vi "project.vi"() -> ()   [LabVIEW 2014]
panel:
  out "Main Valve Position":bool
  out "Motor Running in Delta":bool
  out "Motor Running in Star":bool
  in  "Main Switch Control":bool
  out "Compressor Main Switch":bool
  in  "Boolean":bool
  out "Stage-1 Pressure":u8(slide) scale=0.0..400.0
  out "Inlet Pressure after BDV":u8(slide) scale=0.0..40.0
  out "Inlet\nPressure":u8(slide) scale=0.0..40.0
  out "GD-2 Trend (%LEL)":T1(graph)
  out "GD-1 Trend (%LEL)":T2(graph)
  in  "Low GD-2 %LEL SP":dbl
  in  "High GD-2 %LEL SP":dbl
  in  "Low GD-1 %LEL SP":dbl
  in  "High GD-1 %LEL SP":dbl
  in  "Low Lube Oil Temp SP":dbl
  in  "High Lube Oil Temp SP":dbl
  in  "Low Storage Temp SP":dbl
  in  "High Storage Temp SP":dbl
  in  "Low Stg-3 Temp SP":dbl
  in  "High Stg-3 Temp SP":dbl
  in  "Low Stg-2    Temp SP":dbl
  in  "High Stg-2 Temp SP":dbl
  in  "Low Stg-1 Temp SP":dbl
  in  "High Stg-1 Temp SP":dbl
  in  "Low Inlet Temp SP":dbl
  in  "High Inlet Temp SP":dbl
  in  "Low Lube Oil  Stg-1 Pressure SP":dbl
  in  "High Lube Oil Stg-1 Pressure SP":dbl
  in  "Low Lube Oil Pressure SP":dbl
  in  "High Lube Oil Pressure SP":dbl
  in  "Low Storage Pressure SP":dbl
  in  "High Storage Pressure SP":dbl
  in  "Low Stg-3 Pressure SP 4":dbl
  in  "High Stg-3 Pressure SP":dbl
  in  "Low Stg-2 Pressure SP":dbl
  in  "High Stg-2 Pressure SP":dbl
  in  "Low Stg-1 Pressure SP":dbl
  in  "High Stg-1 Pressure SP":dbl
  in  "Low Inlet Pressure SP":dbl
  in  "High Inlet Pressure SP":dbl
  out "Discharge MFM Flow Rate Trend (Kg/m2)":dbl(graph)
  out "Discharge MFM Total Kg Trend (Kg)":dbl(graph)
  out "Inlet MFM Flow Rate Trend (Kg/m2)":dbl(graph)
  out "Inlet MFM Total Kg Trend (Kg)":dbl(graph)
  out "Lube Oil Temperature Trend (degC)":dbl(graph)
  out "Storage Temperature Trend (degC)":dbl(graph)
  out "Stage-3 Temperature Trend (degC)":dbl(graph)
  out "Stage-2 Temperature Trend (degC)":dbl(graph)
  out "Stage-1 Temperature Trend (degC)":T3(graph)
  out "Inlet Temperature Trend (degC)":T4(graph)
  out "Lube Oil Stage-1 Pressure Trend (Bar) 2":dbl(graph)
  out "Lube Oil Pressure Trend (Bar)":dbl(graph)
  out "Storage Pressure Trend (Bar)":dbl(graph)
  out "Stage-3 Pressure Trend (Bar)":dbl(graph)
  out "Stage-2 Pressure Trend (Bar)":T5(graph)
  out "Stage-1 Pressure Trend (Bar)":T6(graph)
  out "Inlet Pressure after BDV Trend (Bar)":T7(graph)
  out "Inlet Pressure Trend (Bar)":dbl(graph)
  in  "Air Compressor\nstopped/breakdown":bool
  in  "Wire cut":bool
  out "Alarm(s) 4":string
  out "Instrument Air Pressure Gauge (Bar)":dbl(knob) scale=0.0..10.0
  in  "Compressor Start":bool
  out "H":bool
  out "L":bool
  out "H":bool
  out "L":bool
  out "H":bool
  out "L":bool
  out "H":bool
  out "L":bool
  out "H":bool
  out "L":bool
  out "H":bool
  out "L":bool
  out "Alarm(s) 3":string
  out "Alarm(s) 2":string
  out "Lubrication oil Level":dbl(slide) scale=0.0..10.0
  in  "Fill":dbl(slide) scale=0.0..10.0
  out "Alarm(s)":string
  out "CO2 Flooding in Progress":bool
  in  "Fire":bool
  out "Fire Detector-2":bool
  out "Fire Detector-1":bool
  out "Lube Oil Temp":u8(slide) scale=0.0..250.0
  out "Storage Temp":u8(slide) scale=0.0..250.0
  out "Stage-3 \nTemp":u8(slide) scale=0.0..250.0
  out "Stage-2\nTemp":u8(slide) scale=0.0..250.0
  out "Stage-1 \nTemp":u8(slide) scale=0.0..250.0
  out "Inlet\n Temp":u8(slide) scale=0.0..100.0
  out "MFM Flow Rate (Inlet)":dbl
  out "MFM Flow Rate (Discharge)":dbl
  out "MFM Total Kg (Inlet)":dbl format="%#_9g"
  out "MFM Total Kg (Discharge)":dbl format="%#_9g"
  out "Lube oil Stage-1 Pressure":cluster{u8, u8}(slide)={17, 12} scale=0.0..100.0
  out "Lube oil Pressure":cluster{u8, u8}(slide)={17, 12} scale=0.0..10.0
  out "Storage Pressure":cluster{u8, u8}(slide)={17, 12} scale=0.0..400.0
  out "Stage-3 Pressure":cluster{u8, u8}(slide)={17, 12} scale=0.0..400.0
  out "Stage-2 Pressure":cluster{u8, u8}(slide)={17, 12} scale=0.0..400.0
  out "Communication Status":string
  out "Compressor Running Status":string
  # "FIRE SUPPRESSION SAFETY INTERLOCK"
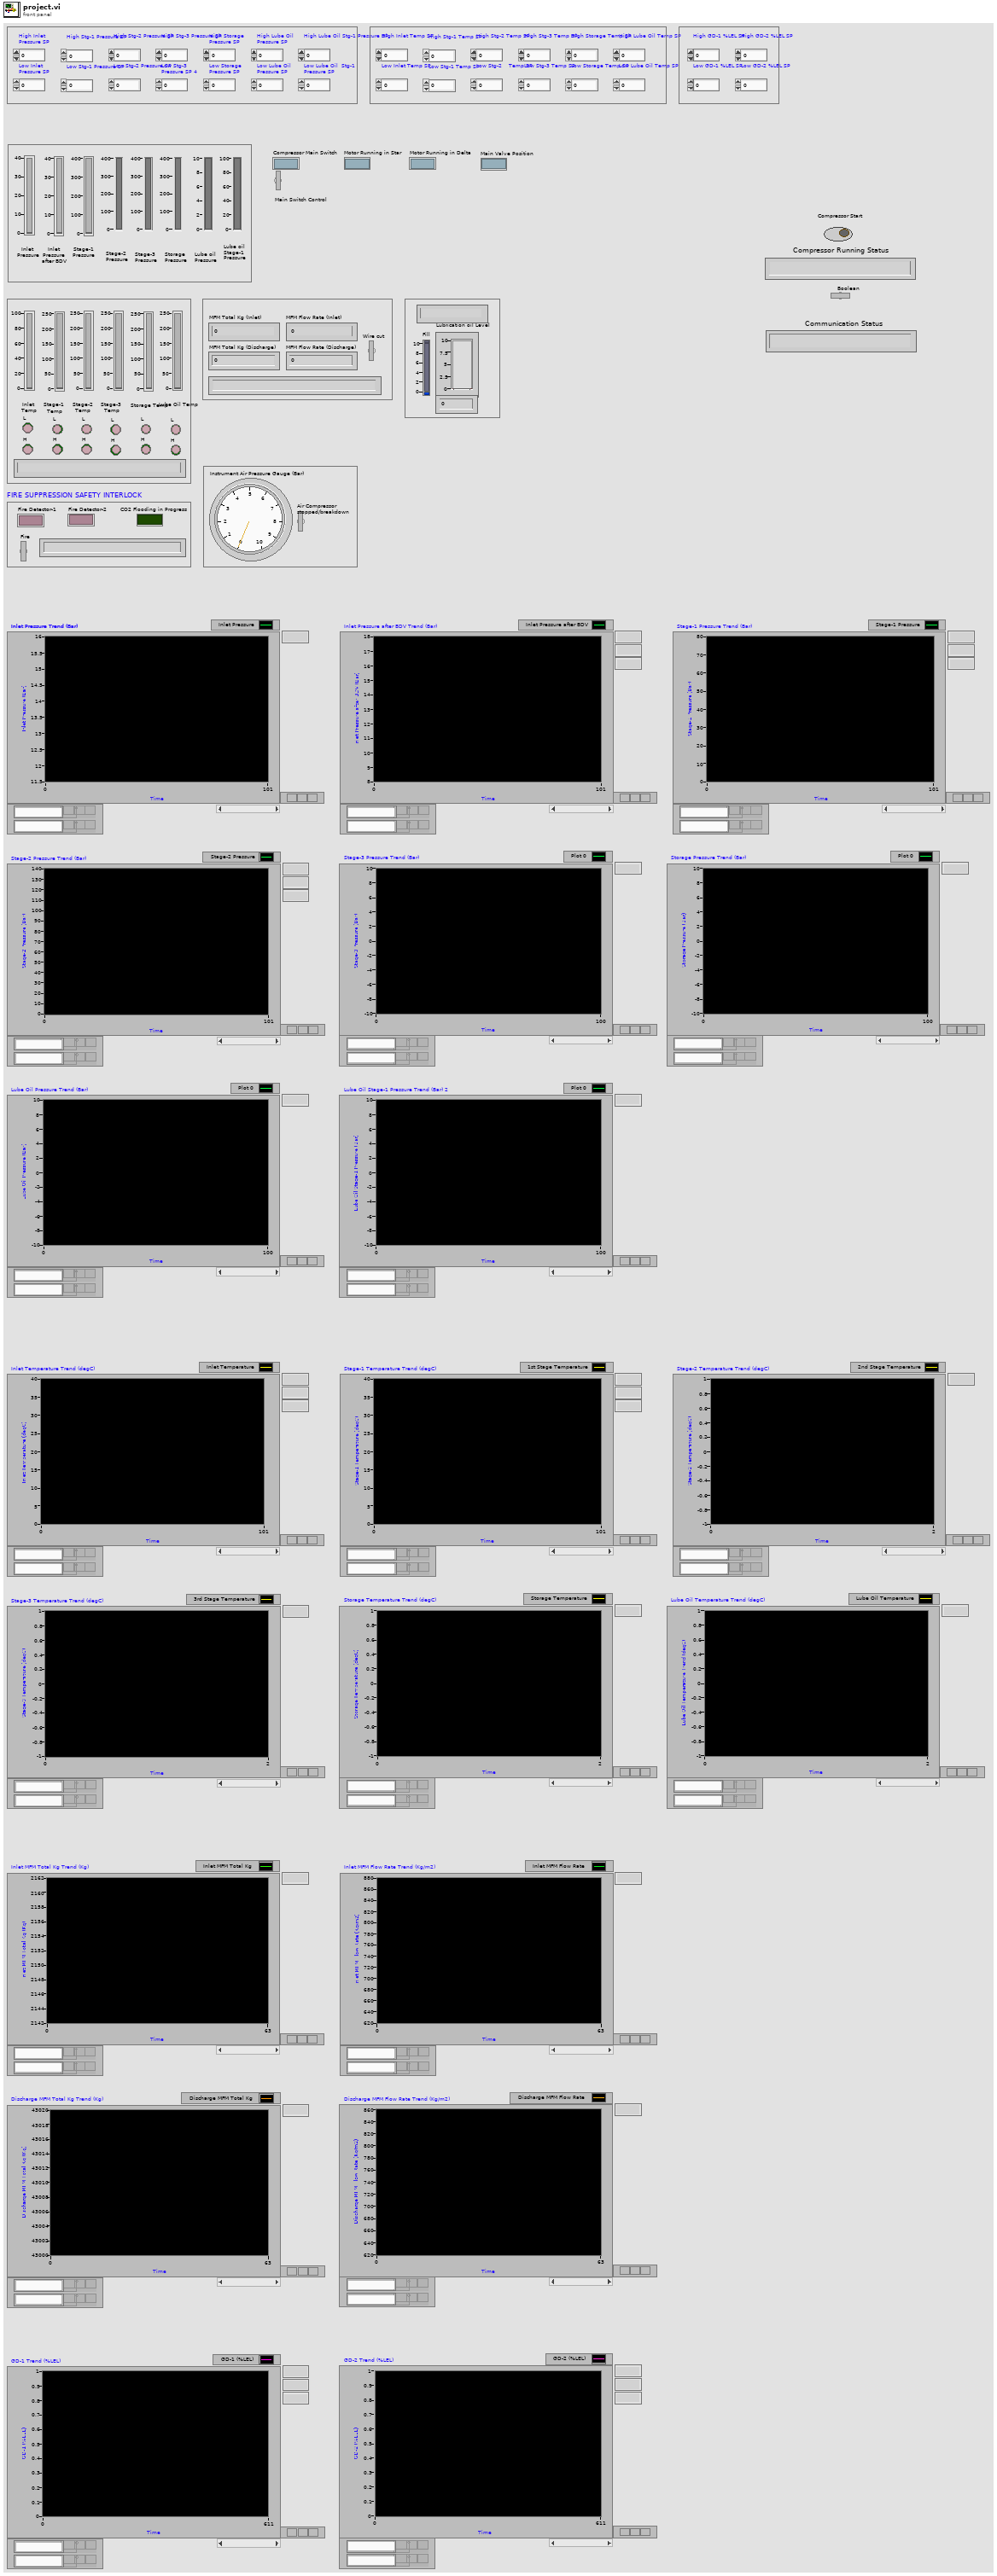
[diagram p1: front panel]
types:
  T1 = cluster{"number: 0 to 1":dbl, "High GD-1 %LEL SP  ":dbl, "Low GD-1 %LEL SP":dbl}
  T2 = cluster{"number: 0 to 1":dbl, "High GD-2 %LEL SP  ":dbl, "Low GD-2 %LEL SP":dbl}
  T3 = cluster{dbl, "High Stg-1 Temp SP":dbl, "Low Stg-1 Temp SP":dbl}
  T4 = cluster{dbl, "High Inlet Temp SP":dbl, "Low Inlet Temp SP":dbl}
  T5 = cluster{dbl, "High Stg-2 Pressure SP":dbl, "Low Stg-2 Pressure SP":dbl}
  T6 = cluster{dbl, "High Stg-1 Pressure SP":dbl, "Low Stg-1 Pressure SP":dbl}
  T7 = cluster{dbl, "High Inlet Pressure SP":dbl, "Low Inlet Pressure SP":dbl}
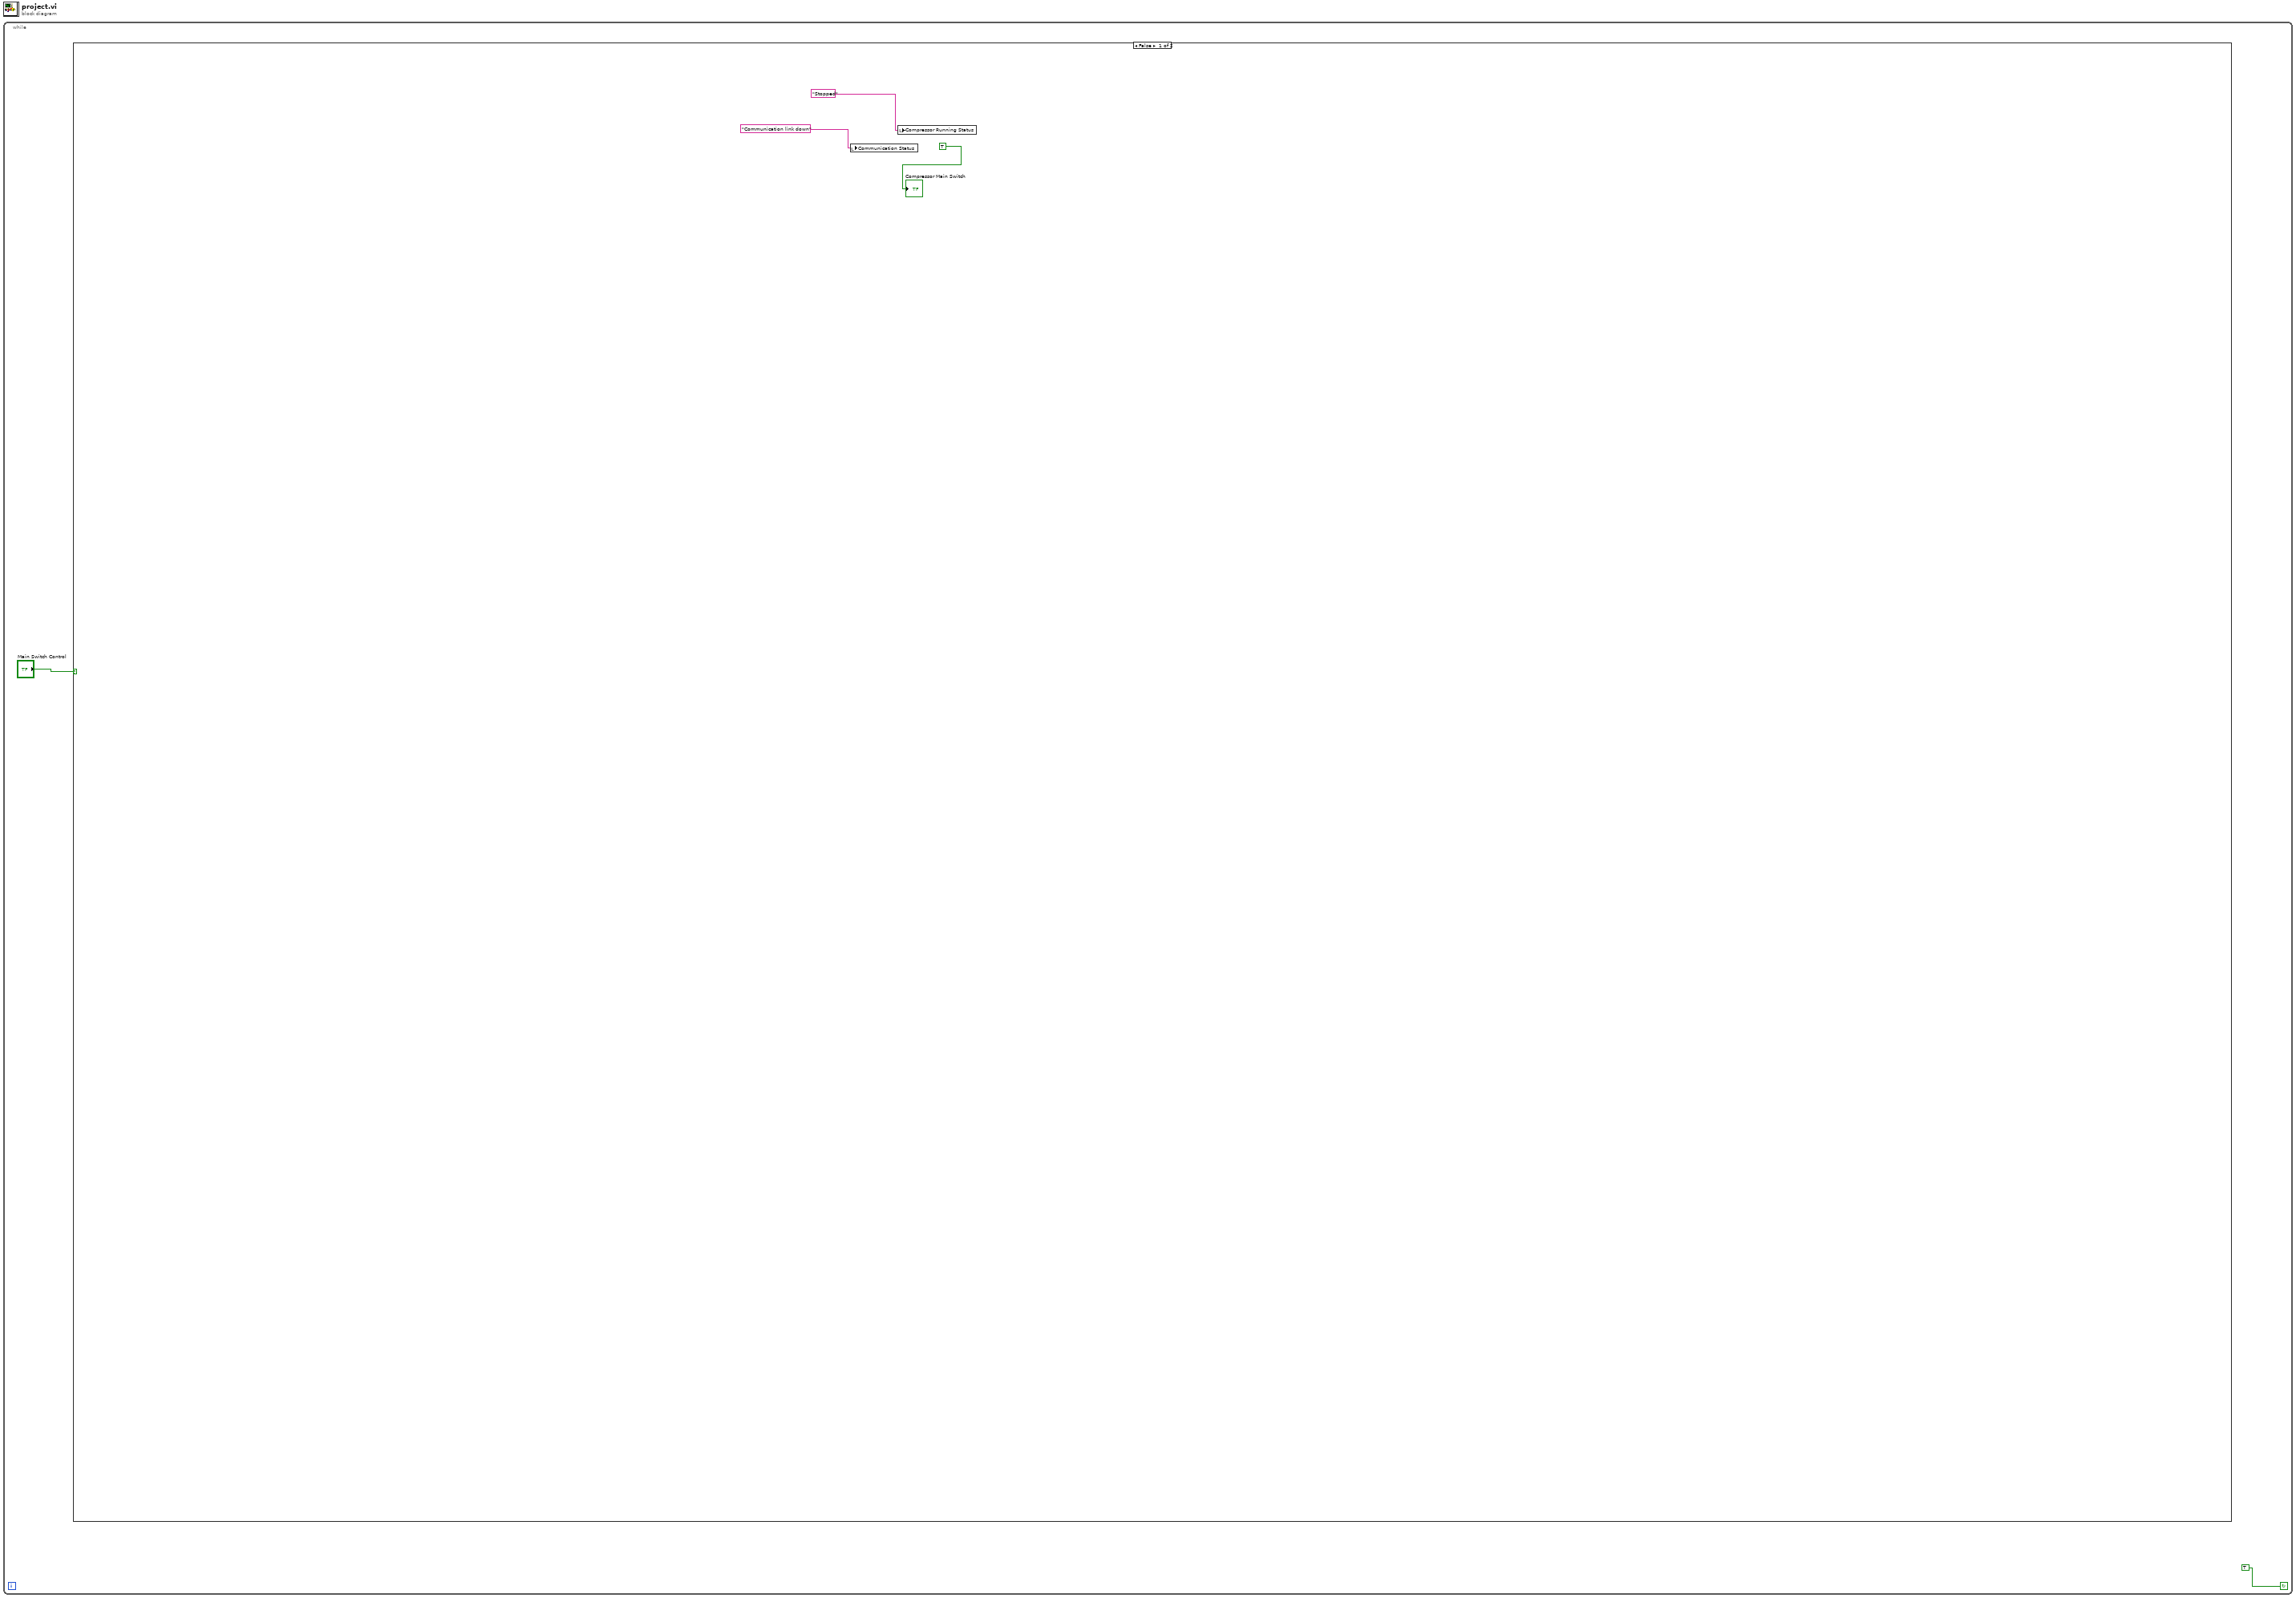
[diagram p0: block diagram]
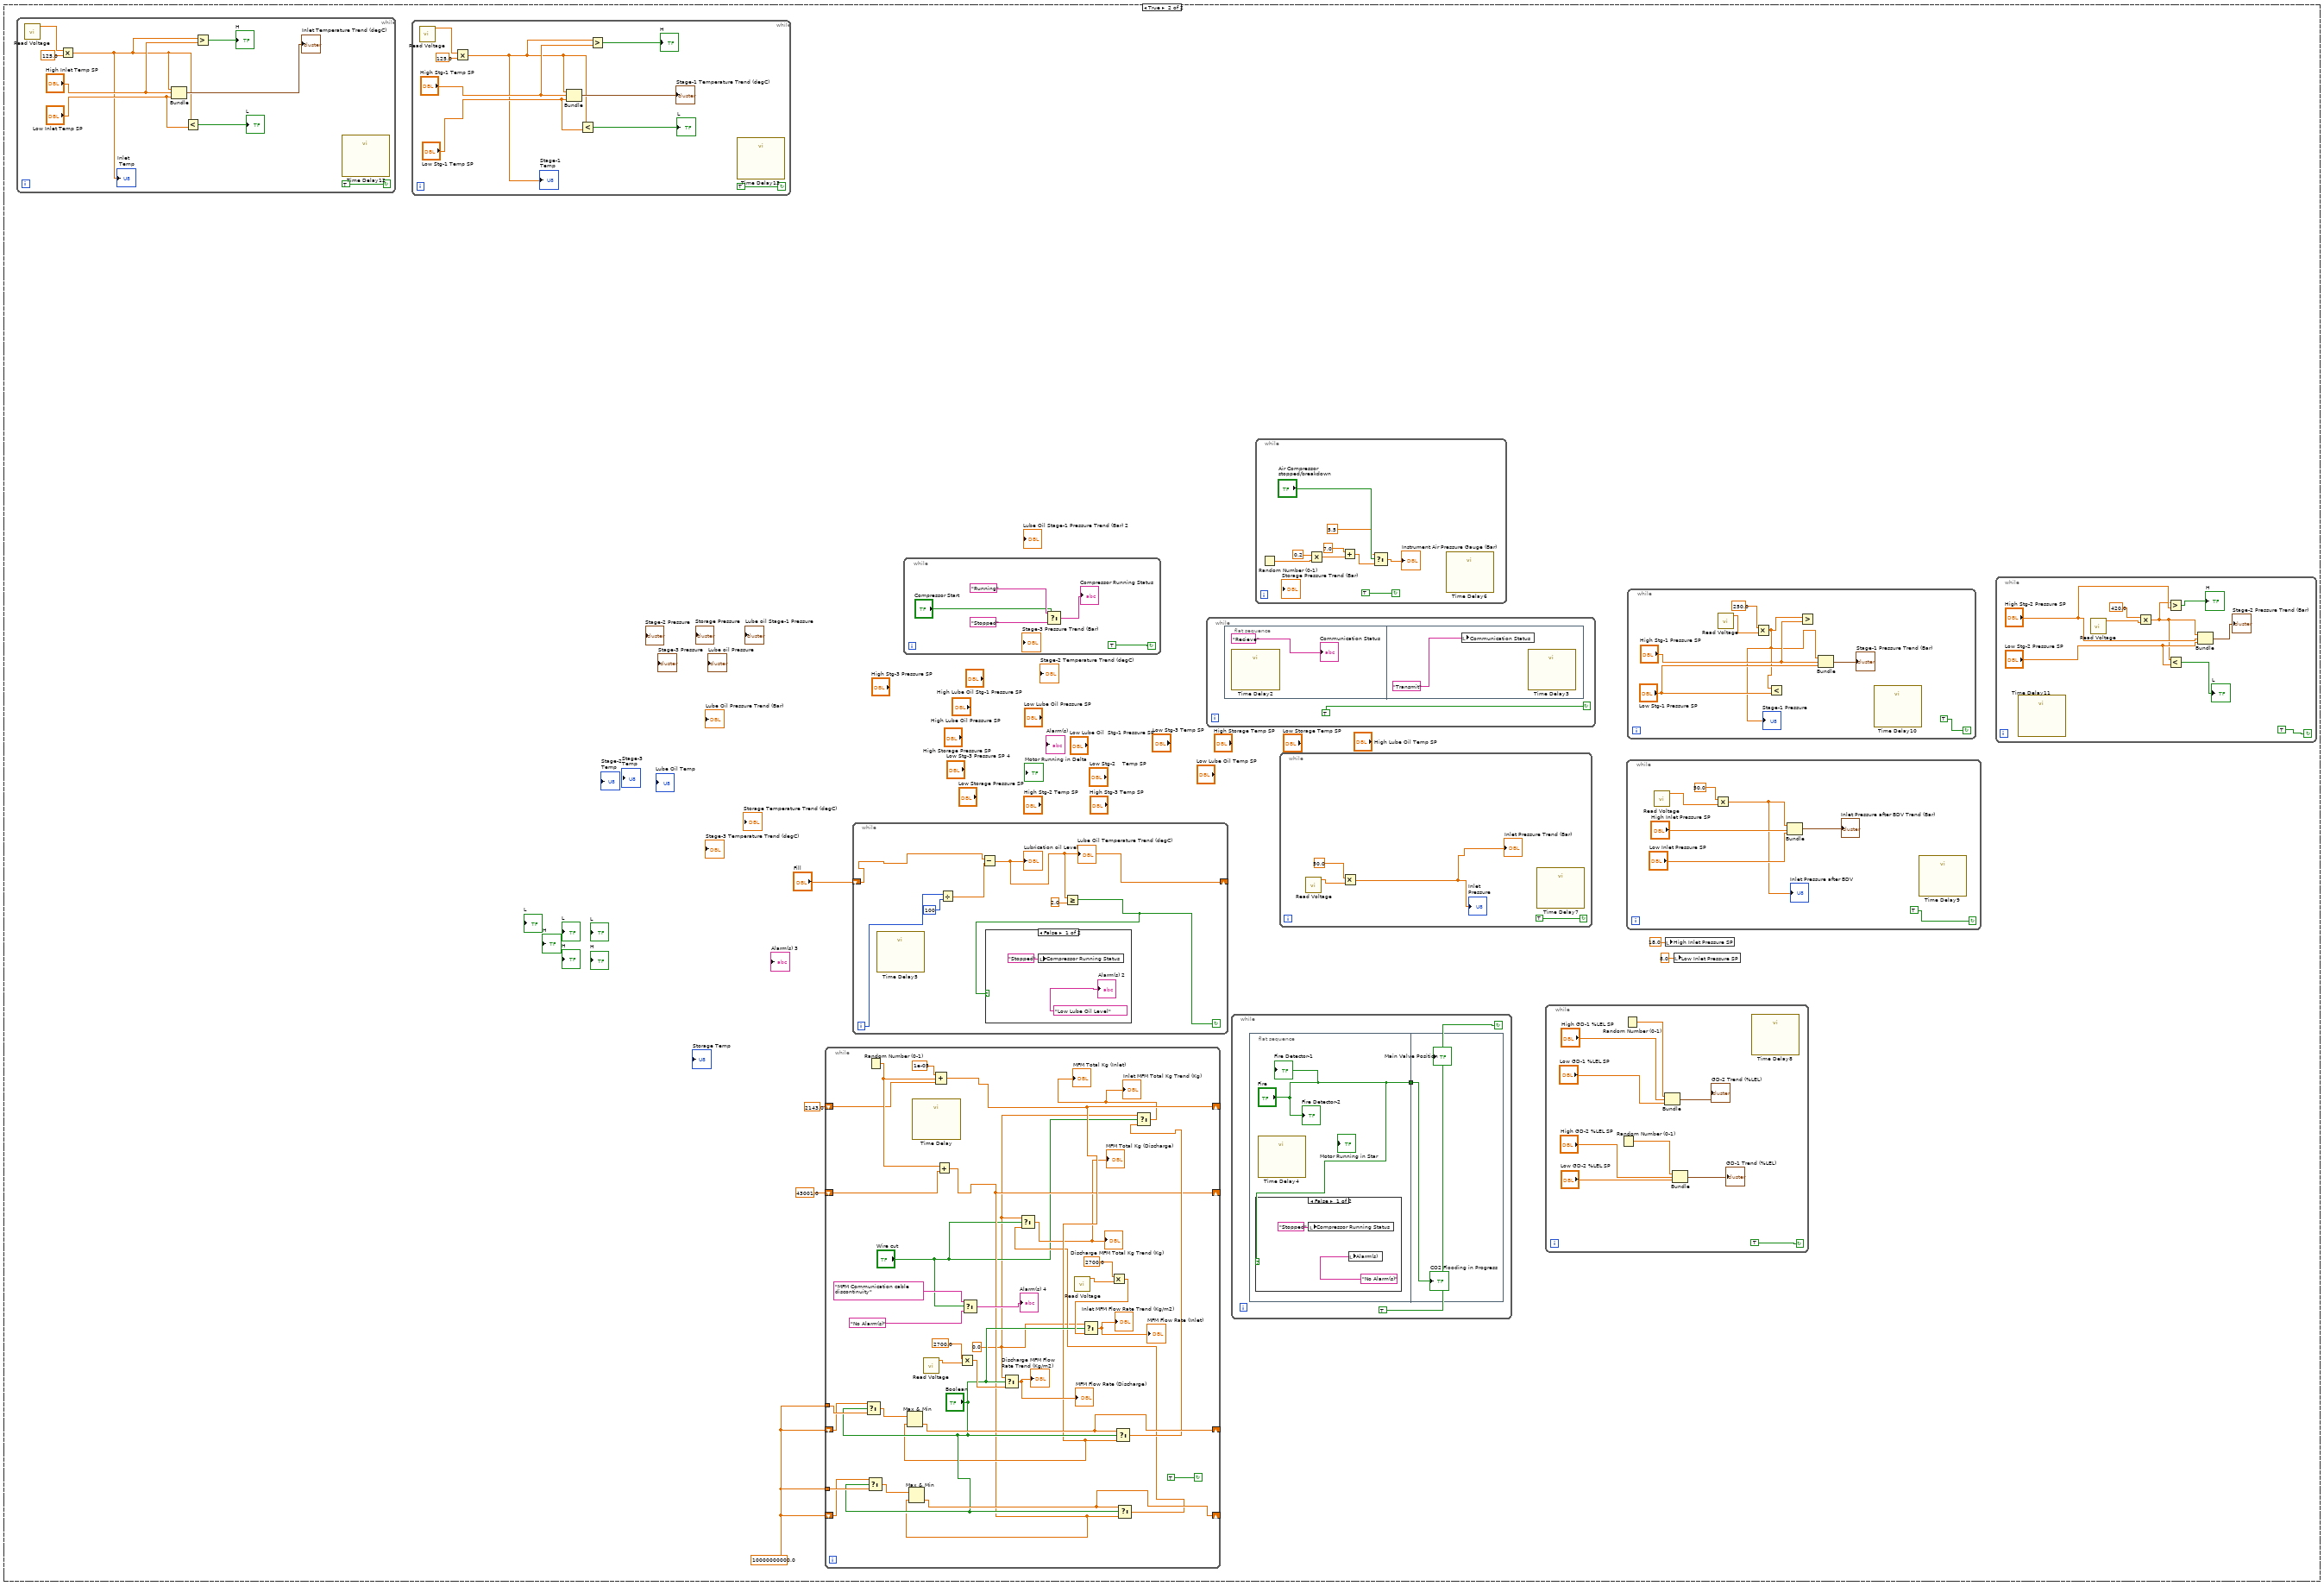
[diagram p2: hidden frame]
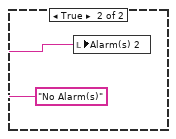
[diagram p3: hidden frame]
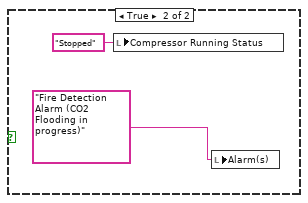
[diagram p4: hidden frame]
diagram:
  n1 = while {
    stop <- TRUE continue-if-true
    n2 = case shown="False" "Main Switch Control" {
      frame False {
        n3 = local write "Communication Status"("Communication link down" ("Compressor Running Status")) -> ()
        n4 = local write "Compressor Running Status"("Stopped" ("Compressor Running Status")) -> ()
        "Compressor Main Switch" <- TRUE
      }
      frame True {
        w6 = 10000000000.0
        n5 = while {
          stop <- TRUE continue-if-true
          n6 = call "Read Voltage.vi"() -> ("voltage"=w28:dbl)  [unwired: 6 in, 1 out]
          n7 = Multiply(x=w28, y=125.0) -> (x*y=w22:dbl)
          "Inlet\n Temp" <- w22
          n8 = Bundle(w22, "High Inlet Temp SP"="High Inlet Temp SP", "Low Inlet Temp SP"="Low Inlet Temp SP") -> (→"Inlet Temperature Trend (degC)":T4)  [unwired: 1 in]
          n9 = Less?(x=w22, y="Low Inlet Temp SP") -> (x < y?=→"L":bool)
          n10 = Greater?(x=w22, y="High Inlet Temp SP") -> (0:→"H":bool)
          n11 = call "Time Delay12"() -> ()  [unwired: 11 in, 1 out]
        }
        n12 = while {
          stop <- TRUE continue-if-true
          n13 = call "Read Voltage.vi"() -> ("voltage"=w19:dbl)  [unwired: 6 in, 1 out]
          n14 = Multiply(x=w19, y=125.0) -> (x*y=w12:dbl)
          "Stage-1 \nTemp" <- w12
          n15 = Bundle(w12, "High Stg-1 Temp SP"="High Stg-1 Temp SP", "Low Stg-1 Temp SP"="Low Stg-1 Temp SP") -> (→"Stage-1 Temperature Trend (degC)":T3)  [unwired: 1 in]
          n16 = Less?(x=w12, y="Low Stg-1 Temp SP") -> (x < y?=→"L":bool)
          n17 = Greater?(x=w12, y="High Stg-1 Temp SP") -> (0:→"H":bool)
          n18 = call "Time Delay13"() -> ()  [unwired: 11 in, 1 out]
        }
        n19 = while {
          shift-right: [w108] -> _
          shift-left: 2143.0 -> [w122]
          shift-right: [w105] -> _
          shift-left: 43001.0 -> [w124]
          shift-right: [w121] -> _
          shift-left: w6 -> [w115]
          tunnel: w6 -> [w119]
          shift-right: [w116] -> _
          shift-left: w6 -> [w114]
          tunnel: w6 -> [w117]
          stop <- TRUE continue-if-true
          w101 = 0.0
          n20 = Select(t=w115, s="Boolean", f=w119) -> (s? t:f=w120:dbl)
          n21 = Select(t=w114, s="Boolean", f=w117) -> (s? t:f=w118:dbl)
          n22 = Random Number (0-1)() -> (number: 0 to 1=w133:dbl)
          n23 = call "Time Delay"() -> ()  [unwired: 11 in, 1 out]
          n24 = call "Read Voltage.vi"() -> ("voltage"=w125:dbl)  [unwired: 6 in, 1 out]
          n25 = Compound Arithmetic op=ADD(1e-05, w133, w122) -> (w108:dbl)
          n26 = Max & Min(x=w120, y=w108) -> (min(x,y)=w121:dbl)  [unwired: 1 out]
          n27 = Add(x=w133, y=w124) -> (x+y=w105:dbl)
          n28 = Max & Min(x=w118, y=w105) -> (min(x,y)=w116:dbl)  [unwired: 1 out]
          n29 = Multiply(x=2700.0, y=w125) -> (x*y=w113:dbl)
          n30 = Select(t="MFM Communication cable discontinuity" ("Compressor Running Status"), s="Wire cut", f="No Alarm(s)" ("Alarm(s)")) -> (s? t:f=→"Alarm(s) 4":string)
          n31 = Select(t=w101, s="Boolean", f=w113) -> (s? t:f=→"Discharge MFM Flow Rate Trend (Kg/m2)" →"MFM Flow Rate (Discharge)":dbl)
          n32 = call "Read Voltage.vi"() -> ("voltage"=w127:dbl)  [unwired: 6 in, 1 out]
          n33 = Multiply(x=2700.0, y=w127) -> (x*y=w112:dbl)
          n34 = Select(t=w101, s="Boolean", f=w112) -> (s? t:f=→"Inlet MFM Flow Rate Trend (Kg/m2)" →"MFM Flow Rate (Inlet)":dbl)
          n35 = Select(t=w121, s="Boolean", f=w108) -> (s? t:f=w106:dbl)
          n36 = Select(t=w116, s="Boolean", f=w105) -> (s? t:f=w104:dbl)
          n37 = Select(t=w101, s="Wire cut", f=w104) -> (s? t:f=→"Discharge MFM Total Kg Trend (Kg)" →"MFM Total Kg (Discharge)":dbl)
          n38 = Select(t=w101, s="Wire cut", f=w106) -> (s? t:f=→"MFM Total Kg (Inlet)" →"Inlet MFM Total Kg Trend (Kg)":dbl)
        }
        n39 = while {
          shift-right: [w72] -> _
          shift-left: "Fill" -> [w74]
          i -> [w73]
          stop <- w71 continue-if-true
          n40 = call "Time Delay5"() -> ()  [unwired: 11 in, 1 out]
          n41 = Divide(x=w73, y=100) -> (x/y=w76:dbl)
          n42 = Subtract(x=w74, y=w76) -> (x-y=w72:dbl)
          "Lubrication oil Level" <- w72
          n43 = Greater Or Equal?(x=w72, y=2.0) -> (x >= y?=w71:bool)
          n44 = case shown="False" w71 {
            frame False {
              n45 = local write "Compressor Running Status"("Stopped" ("Compressor Running Status")) -> ()
              "Alarm(s) 2" <- "Low Lube Oil Level" ("Alarm(s)")
            }
            frame True {
              n46 = local write "Alarm(s) 2"("No Alarm(s)" ("Alarm(s)")) -> ()
            }
          }
        }
        n47 = while {
          stop <- TRUE continue-if-true
          n48 = Select(t="Running" ("Compressor Running Status"), s="Compressor Start", f="Stopped" ("Compressor Running Status")) -> (s? t:f=→"Compressor Running Status":string)
        }
        n49 = while {
          stop <- TRUE continue-if-true
          n50 = flat-sequence {
            frame #0 {
              n51 = call "Time Delay2"() -> ()  [unwired: 11 in, 1 out]
              "Communication Status" <- "Recieve" ("Communication Status")
            }
            frame #1 {
              n52 = local write "Communication Status"("Transmit" ("Communication Status")) -> ()
              n53 = call "Time Delay3"() -> ()  [unwired: 11 in, 1 out]
            }
          }
        }
        n54 = while {
          stop <- TRUE continue-if-true
          n55 = flat-sequence {
            tunnel: ["Fire"] -> w82
            tunnel: w82 -> [w88]
            frame #0 {
              n56 = case shown="False" "Fire" {
                frame False {
                  n57 = local write "Compressor Running Status"("Stopped" ("Compressor Running Status")) -> ()
                  n58 = local write "Alarm(s)"("No Alarm(s)" ("Alarm(s)")) -> ()
                }
                frame True {
                  n59 = local write "Compressor Running Status"("Stopped" ("Compressor Running Status")) -> ()
                  n60 = local write "Alarm(s)"("Fire Detection Alarm (CO2 Flooding in progress)" ("Alarm(s)")) -> ()
                }
              }
              n61 = call "Time Delay4"() -> ()  [unwired: 11 in, 1 out]
              "Fire Detector-1" <- "Fire"
              "Fire Detector-2" <- "Fire"
            }
            frame #1 {
              "CO2 Flooding in Progress" <- w88
            }
          }
        }
        n62 = while {
          stop <- TRUE continue-if-true
          n63 = Random Number (0-1)() -> (number: 0 to 1=w64:dbl)
          n64 = Multiply(x=0.2, y=w64) -> (x*y=w62:dbl)
          n65 = Add(x=7.0, y=w62) -> (x+y=w59:dbl)
          n66 = Select(t=5.5, s="Air Compressor\nstopped/breakdown", f=w59) -> (s? t:f=→"Instrument Air Pressure Gauge (Bar)":dbl)
          n67 = call "Time Delay6"() -> ()  [unwired: 11 in, 1 out]
        }
        n68 = while {
          stop <- TRUE continue-if-true
          n69 = call "Read Voltage.vi"() -> ("voltage"=w54:dbl)  [unwired: 6 in, 1 out]
          n70 = Multiply(x=50.0, y=w54) -> (x*y=→"Inlet Pressure Trend (Bar)" →"Inlet\nPressure":dbl)
          n71 = call "Time Delay7"() -> ()  [unwired: 11 in, 1 out]
        }
        n72 = while {
          stop <- TRUE continue-if-true
          n73 = Random Number (0-1)() -> (number: 0 to 1=w44:dbl)
          n74 = Random Number (0-1)() -> (number: 0 to 1=w49:dbl)
          n75 = Bundle("number: 0 to 1"=w49, "High GD-1 %LEL SP"="High GD-1 %LEL SP", "Low GD-1 %LEL SP"="Low GD-1 %LEL SP") -> (→"GD-2 Trend (%LEL)":T1)  [unwired: 1 in]
          n76 = Bundle("number: 0 to 1"=w44, "High GD-2 %LEL SP"="High GD-2 %LEL SP", "Low GD-2 %LEL SP"="Low GD-2 %LEL SP") -> (→"GD-1 Trend (%LEL)":T2)  [unwired: 1 in]
          n77 = call "Time Delay8"() -> ()  [unwired: 11 in, 1 out]
        }
        n78 = while {
          stop <- TRUE continue-if-true
          n79 = call "Read Voltage.vi"() -> ("voltage"=w42:dbl)  [unwired: 6 in, 1 out]
          n80 = Multiply(x=50.0, y=w42) -> (x*y=w37:dbl)
          "Inlet Pressure after BDV" <- w37
          n81 = Bundle(w37, "High Inlet Pressure SP"="High Inlet Pressure SP", "Low Inlet Pressure SP"="Low Inlet Pressure SP") -> (→"Inlet Pressure after BDV Trend (Bar)":T7)  [unwired: 1 in]
          n82 = call "Time Delay9"() -> ()  [unwired: 11 in, 1 out]
        }
        n83 = while {
          stop <- TRUE continue-if-true
          n84 = call "Read Voltage.vi"() -> ("voltage"=w35:dbl)  [unwired: 6 in, 1 out]
          n85 = Multiply(x=250.0, y=w35) -> (x*y=w30:dbl)
          "Stage-1 Pressure" <- w30
          n86 = Less?(x=w30, y="Low Stg-1 Pressure SP") -> ()  [unwired: 1 out]
          n87 = Greater?(x=w30, y="High Stg-1 Pressure SP") -> ()  [unwired: 1 out]
          n88 = Bundle(w30, "High Stg-1 Pressure SP"="High Stg-1 Pressure SP", "Low Stg-1 Pressure SP"="Low Stg-1 Pressure SP") -> (→"Stage-1 Pressure Trend (Bar)":T6)  [unwired: 1 in]
          n89 = call "Time Delay10"() -> ()  [unwired: 11 in, 1 out]
        }
        n90 = local write "High Inlet Pressure SP"(18.0 ("High Inlet Pressure SP")) -> ()
        n91 = local write "Low Inlet Pressure SP"(8.0 ("Low Inlet Pressure SP")) -> ()
        n92 = while {
          stop <- TRUE continue-if-true
          n93 = call "Time Delay11"() -> ()  [unwired: 11 in, 1 out]
          n94 = call "Read Voltage.vi"() -> ("voltage"=w97:dbl)  [unwired: 6 in, 1 out]
          n95 = Multiply(x=420.0, y=w97) -> (x*y=w92:dbl)
          n96 = Greater?(x=w92, y="High Stg-2 Pressure SP") -> (0:→"H":bool)
          n97 = Less?(x=w92, y="Low Stg-2 Pressure SP") -> (x < y?=→"L":bool)
          n98 = Bundle(w92, "High Stg-2 Pressure SP"="High Stg-2 Pressure SP", "Low Stg-2 Pressure SP"="Low Stg-2 Pressure SP") -> (→"Stage-2 Pressure Trend (Bar)":T5)  [unwired: 1 in]
        }
      }
    }
  }
